vi "Parse Cats.vi"(8 "error in (no error)":errorcluster, 11 "path to XML document":path=path "C:/Users/frmausse/Desktop/Summer Projects/VIStore (Actor)/Source/StoreCats.xml") -> (0 "error out":errorcluster, 3 "Categories":refnum<class "Category.lvclass">[](array[class]))   [LabVIEW 2015, in "Category Library.lvlib" / "Category.lvclass"]
uses:
  Category.lvclass
  Category.lvclass/Category.ctl
  <vilib>/xml/Load XML File.vi
  <vilib>/xml/Close Reference(Node).vi
  <vilib>/xml/NI_XML.lvlib
  <resource>/objmgr/DOMUserDefRef.rc
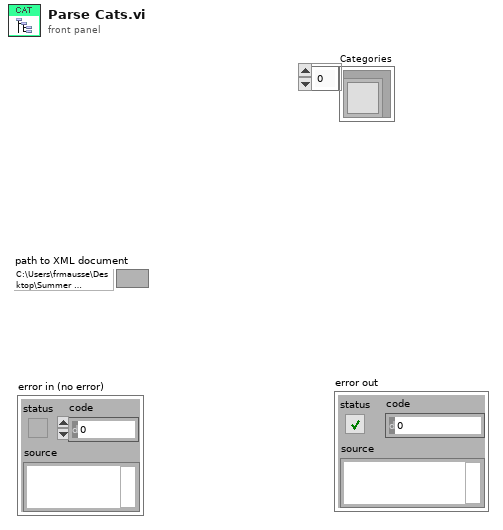
[diagram p1: front panel]
types:
  T1 = typedef "imagedata.ctl" = cluster{"image type":i32, "image depth":i32, "image":u8[], "mask":u8[], "colors":u32[], "Rectangle":cluster{"left":i16, "top":i16, "right":i16, "bottom":i16}}
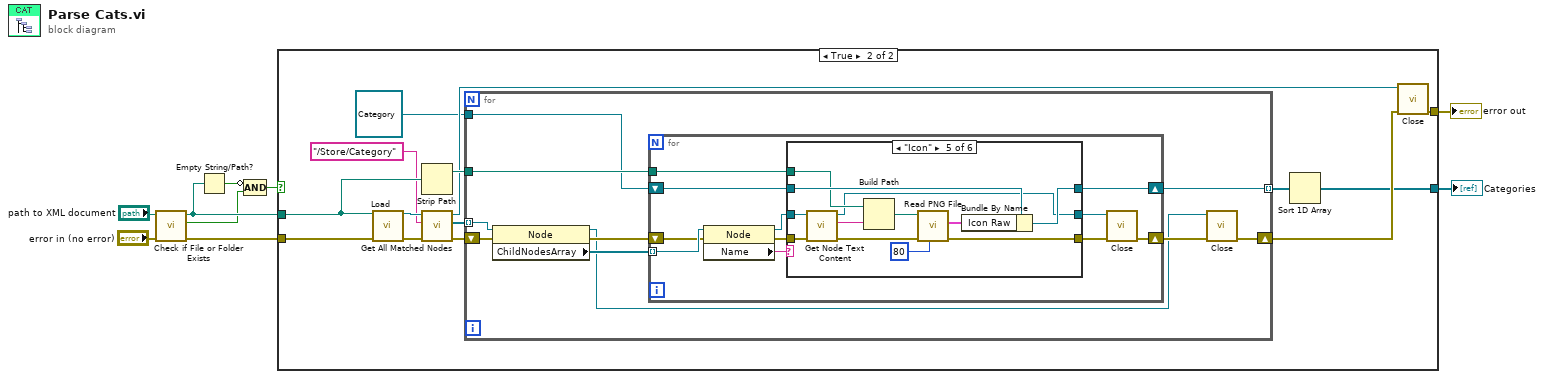
[diagram p0: block diagram]
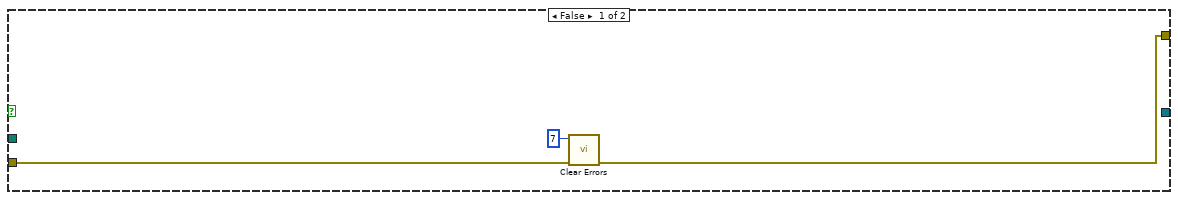
[diagram p2: hidden frame]
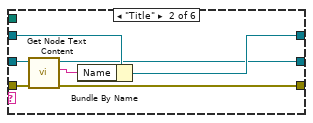
[diagram p4: hidden frame]
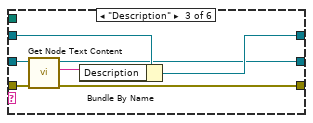
[diagram p5: hidden frame]
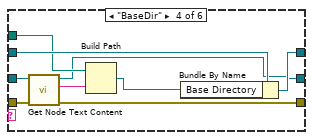
[diagram p6: hidden frame]
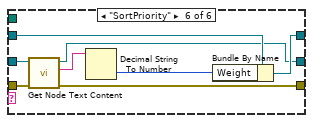
[diagram p7: hidden frame]
diagram:
  n1 = call <vilib>:"Check if File or Folder Exists.vi"("error in (no error)"="error in (no error)", "path"="path to XML document") -> ("error out"=w5:errorcluster, "file or folder exists?"=w2:bool, "dup path"=w4:path)  [unwired: 7 in]
  n2 = Empty String/Path?(string/path=w4) -> (empty?=w3:bool)
  n3 = Compound Arithmetic op=AND(invert w3, w2) -> (w1:bool)
  n4 = case shown="True" w1 {
    tunnel: w4 -> [_ w26]
    tunnel: [w10 w17] -> w9
    tunnel: w5 -> [w12 w16]
    tunnel: [_ w13] -> w8
    frame False {
      n5 = call <vilib>:"Clear Errors.vi"("error in (no error)"=w12, "specific error code to clear (0: all)"=7) -> ("error out"=w10:errorcluster)  [unwired: 4 in, 1 out]
    }
    frame True {
      n6 = call-poly <vilib>:"Load.vi"("path to XML document"=w26, "error in (no error)"=w16) -> ("DOM document out"=w22:refnum<k20>, "error out"=w23:errorcluster)  [unwired: 11 in, 1 out]
      n7 = Strip Path(path=w26) -> (stripped path=w25:path)  [unwired: 1 out]
      n8 = call <vilib>:"Get All Matched Nodes.vi"("error in (no error)"=w23, "XPath expression"="/Store/Category" ("Tag Name"), "node in"=w22) -> ("error out"=w18:errorcluster, "node result array"=w19:refnum<k20>[], "node out"=w20:refnum<k20>)  [unwired: 6 in]
      n9 = for {
        tunnel: [w36] -> w14 mode=indexing
        tunnel: w25 -> [w35]
        tunnel: w19 -> [w31] mode=indexing
        shift-right: [w28] -> w24
        shift-left: w18 -> [w30]
        tunnel: refnum<class "Category.lvclass"> refnum ("Category.lvclass") -> [w27]
        n10 = property class="Node"(reference=w31, error in=w30) -> (reference out=w29:refnum<k20>, error out=w33:errorcluster, "ChildNodesArray"=w34:refnum<k20>[])
        n11 = for {
          tunnel: w34 -> [w44] mode=indexing
          shift-right: [w46] -> w36
          shift-left: w27 -> [w47]
          tunnel: w35 -> [w45]
          shift-right: [w38] -> w32
          shift-left: w33 -> [w41]
          n12 = property class="Node"(reference=w44, error in=w41) -> (reference out=w43:refnum<k20>, error out=w42:errorcluster, "Name"=w40:string)
          n13 = case shown="\"Icon\"" w40 {
            tunnel: w47 -> [w50 w57 w64 w73 w85 w93]
            tunnel: [w50 w56 w63 w72 w84 w92] -> w46
            tunnel: w45 -> [_ _ _ w71 w83 _]
            tunnel: w43 -> [w49 w55 w62 w69 w82 w91]
            tunnel: [w49 w53 w61 w67 w80 w89] -> w37
            tunnel: [w48 w51 w59 w65 w77 w88] -> w39
            tunnel: w42 -> [w48 w52 w60 w66 w79 w87]
            frame Default {
            }
            frame "Title" {
              n14 = call <vilib>:"Get Node Text Content.vi"("error in (no error)"=w52, "node in"=w55) -> ("error out"=w51:errorcluster, "node text"=w54:string, "node out"=w53:refnum<k20>)  [unwired: 7 in]
              n15 = Bundle By Name(cluster=w57, "Name"=w54) -> (w56:refnum<class "Category.lvclass">)
            }
            frame "Description" {
              n16 = call <vilib>:"Get Node Text Content.vi"("error in (no error)"=w60, "node in"=w62) -> ("error out"=w59:errorcluster, "node text"=w58:string, "node out"=w61:refnum<k20>)  [unwired: 7 in]
              n17 = Bundle By Name(cluster=w64, "Description"=w58) -> (w63:refnum<class "Category.lvclass">)
            }
            frame "BaseDir" {
              n18 = call <vilib>:"Get Node Text Content.vi"("error in (no error)"=w66, "node in"=w69) -> ("error out"=w65:errorcluster, "node text"=w68:string, "node out"=w67:refnum<k20>)  [unwired: 7 in]
              n19 = Build Path(base path=w71, name or relative path=w68) -> (appended path=w70:path)
              n20 = Bundle By Name(cluster=w73, "Base Directory"=w70) -> (w72:refnum<class "Category.lvclass">)
            }
            frame "Icon" {
              n21 = call <vilib>:"Get Node Text Content.vi"("error in (no error)"=w79, "node in"=w82) -> ("error out"=w78:errorcluster, "node text"=w81:string, "node out"=w80:refnum<k20>)  [unwired: 7 in]
              n22 = Build Path(base path=w83, name or relative path=w81) -> (appended path=w76:path)
              n23 = call <vilib>:"Read PNG File.vi"("Transparency Thresh"=u8 80, "error in (no error)"=w78, "path to PNG file"=w76) -> ("error out"=w77:errorcluster, "image data"=w75:T1)  [unwired: 6 in, 1 out]
              n24 = Bundle By Name(cluster=w85, "Icon Raw"=w75) -> (w84:refnum<class "Category.lvclass">)
            }
            frame "SortPriority" {
              n25 = call <vilib>:"Get Node Text Content.vi"("error in (no error)"=w87, "node in"=w91) -> ("error out"=w88:errorcluster, "node text"=w90:string, "node out"=w89:refnum<k20>)  [unwired: 7 in]
              n26 = Decimal String To Number(string=w90) -> (number=w86:i32)  [unwired: 2 in, 1 out]
              n27 = Bundle By Name(cluster=w93, "Weight"=w86) -> (w92:refnum<class "Category.lvclass">)
            }
          }
          n28 = call-poly <vilib>:"Close.vi"("error in (no error)"=w39, "node"=w37) -> ("error out"=w38:errorcluster)  [unwired: 7 in]
        }
        n29 = call-poly <vilib>:"Close.vi"("error in (no error)"=w32, "node"=w29) -> ("error out"=w28:errorcluster)  [unwired: 7 in]
      }
      n30 = Sort 1D Array(array=w14) -> (sorted array=w13:refnum<class "Category.lvclass">[])
      n31 = call-poly <vilib>:"Close.vi"("error in (no error)"=w24, "node"=w20) -> ("error out"=w17:errorcluster)  [unwired: 7 in]
    }
  }
  "error out" <- w9
  "Categories" <- w8
